vi "main.vi"() -> ()   [LabVIEW 2021]
panel:
  in  "Cancel order":bool
  out "Notification":string
  out "Credit":dbl
  in  "20 Kč":bool
  in  "10 Kč":bool
  in  "5 Kč":bool
  in  "2 Kč":bool
  in  "1 Kč":bool
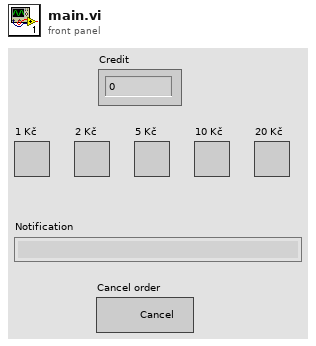
[diagram p1: front panel]
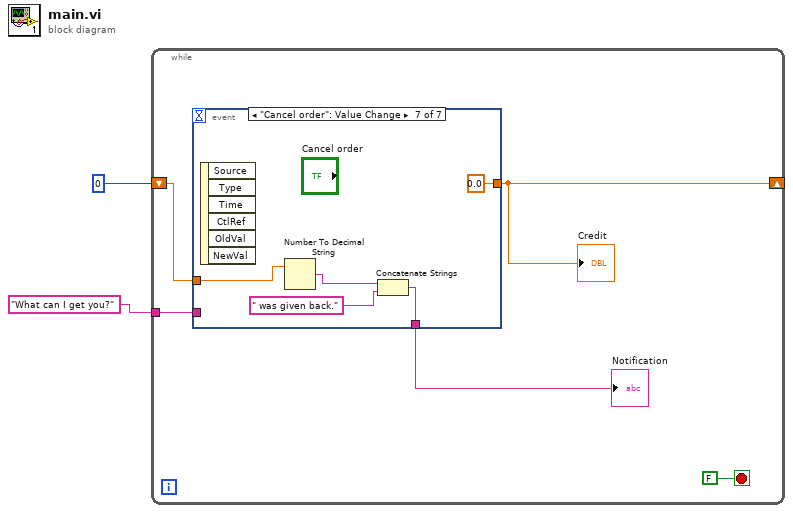
[diagram p0: block diagram]
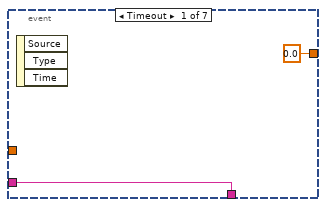
[diagram p2: hidden frame]
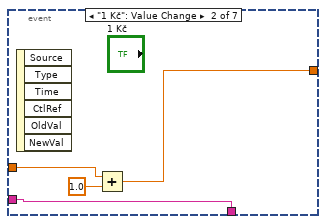
[diagram p3: hidden frame]
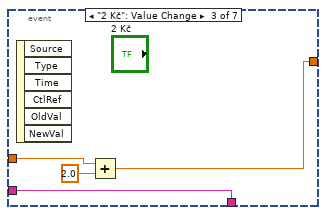
[diagram p4: hidden frame]
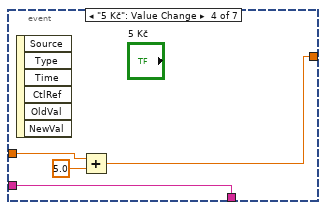
[diagram p5: hidden frame]
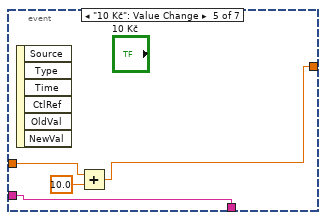
[diagram p6: hidden frame]
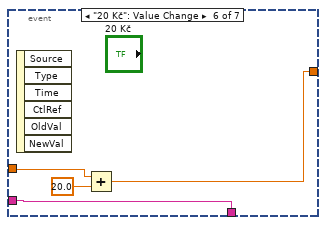
[diagram p7: hidden frame]
diagram:
  n1 = while {
    shift-right: [w5] -> _
    shift-left: 0 -> [w6]
    tunnel: "What can I get you?" -> [w4]
    stop <- FALSE stop-if-true
    n2 = event shown="[6] \"Cancel order\": Value Change" {
      selector: _ -> [_ _ _ _ _ _ _]
      dyn-events: _ -> [_ _ _ _ _ _ _]
      timeout: _ -> [_ _ _ _ _ _ _]
      tunnel: w6 -> [_ w12 w16 w20 w24 w28 w32]
      tunnel: [0.0 w11 w15 w19 w23 w27 0.0] -> w5
      tunnel: [w8 w10 w14 w18 w22 w26 w30] -> w3
      tunnel: w4 -> [w8 w10 w14 w18 w22 w26 _]
      event Timeout {
        n3 = event-data() -> ()  [unwired: 1 in, 3 out]
      }
      event "1 Kč": Value Change {
        n4 = event-data() -> ()  [unwired: 1 in, 6 out]
        n5 = Add(x=w12, y=1.0) -> (x+y=w11:dbl)
      }
      event "2 Kč": Value Change {
        n6 = event-data() -> ()  [unwired: 1 in, 6 out]
        n7 = Add(x=w16, y=2.0) -> (x+y=w15:dbl)
      }
      event "5 Kč": Value Change {
        n8 = event-data() -> ()  [unwired: 1 in, 6 out]
        n9 = Add(x=w20, y=5.0) -> (x+y=w19:dbl)
      }
      event "10 Kč": Value Change {
        n10 = event-data() -> ()  [unwired: 1 in, 6 out]
        n11 = Add(x=w24, y=10.0) -> (x+y=w23:dbl)
      }
      event "20 Kč": Value Change {
        n12 = event-data() -> ()  [unwired: 1 in, 6 out]
        n13 = Add(x=w28, y=20.0) -> (x+y=w27:dbl)
      }
      event "Cancel order": Value Change {
        n14 = event-data() -> ()  [unwired: 1 in, 6 out]
        n15 = Number To Decimal String(number=w32) -> (decimal integer string=w31:string)  [unwired: 1 in]
        n16 = Concatenate Strings(w31, " was given back.") -> (w30:string)
      }
    }
    "Credit" <- w5
    "Notification" <- w3
  }
